vi "vlcTransmitter.vi"(9 "pulse duration":i32=5, 10 "M":i32=16, 11 "Array in":u16[](array[numeric])) -> (1 "Array out":cdb[](array[numeric]), 2 "size(s)":i32)   [LabVIEW 2017]
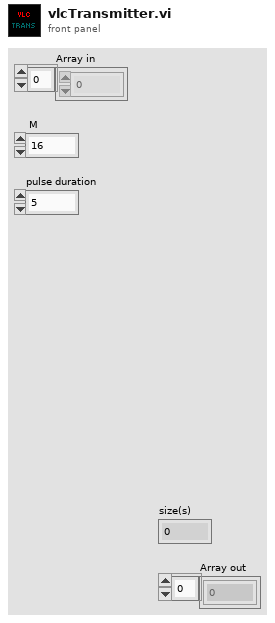
[diagram p1: front panel]
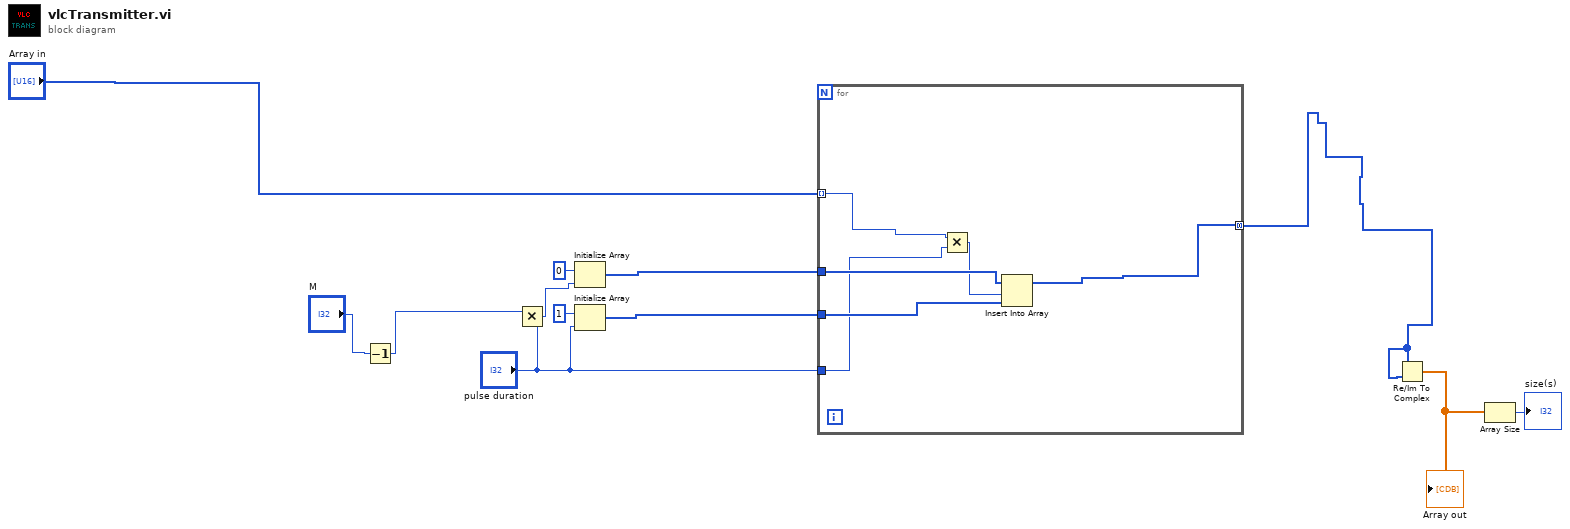
[diagram p0: block diagram]
diagram:
  n1 = Decrement(x="M") -> (x-1=w2:i32)
  n2 = Multiply(x=w2, y="pulse duration") -> (x*y=w8:i32)
  n3 = Initialize Array(0 ("element"), w8) -> (w3:i32[])
  n4 = Initialize Array(1 ("element"), "pulse duration") -> (w4:i32[])
  n5 = for {
    tunnel: w3 -> [w18]
    tunnel: w4 -> [w17]
    tunnel: [w16] -> w9 mode=concatenating
    tunnel: "Array in" -> [w15] mode=indexing
    tunnel: "pulse duration" -> [w14]
    n6 = Multiply(x=w15, y=w14) -> (x*y=w13:i32)
    n7 = Insert Into Array(array=w18, index=w13, new element=w17) -> (w16:i32[])
  }
  n8 = Re/Im To Complex(1:w9, 2:w9) -> (0:w10:cdb[])
  "Array out" <- w10
  n9 = Array Size(array=w10) -> (size(s)=→"size(s)":i32)
